vi "write default value String.vi"(8 "error in":errorcluster, 10 "default value":string, 11 "system tag in":refnum<class "tag descriptor.lvclass">) -> (0 "error out":errorcluster, 3 "system tag out":refnum<class "tag descriptor.lvclass">)   [LabVIEW 2013, in "tag bus.lvlib" / "tag descriptor.lvclass"]
doc: "Converts the provided default value into a string and stores that as the raw default value within the tag."
uses:
  tag descriptor.lvclass
  Data Type.ctl
  tag descriptor.lvclass/tag descriptor.ctl
  tag bus.lvlib
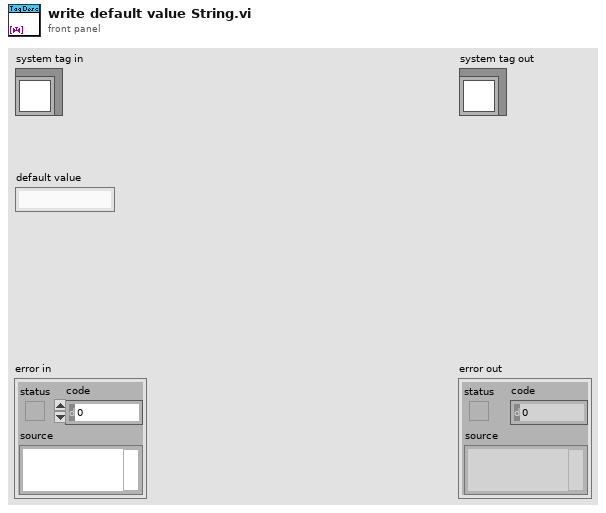
[diagram p1: front panel]
types:
  T1 = typedef "tag bus.lvlib/tag descriptor.lvclass/Data Type.ctl" = enum16{"Double", "Single", "I64", "I32", "I16", "I8", "U64", "U32", "U16", "U8", "Boolean", "String", "Array of Double", "Array of Single", "Array of I64", "Array of I32", "Array of I16", "Array of I8", "Array of U64", "Array of U32", "Array of U16", "Array of U8", "Array of Boolean", "Array of String"}
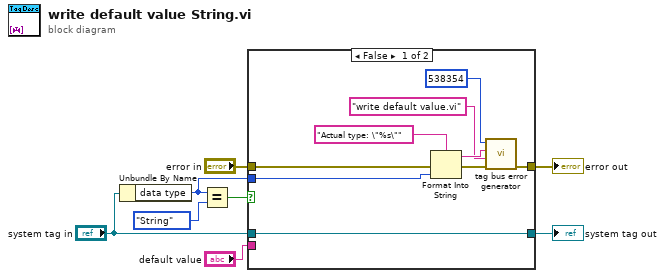
[diagram p0: block diagram]
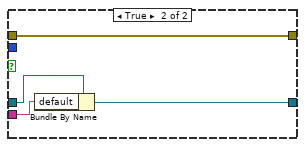
[diagram p2: hidden frame]
diagram:
  n1 = Unbundle By Name("system tag in") -> ("data type"=w4:T1)
  n2 = Equal?(x=w4, y=Data_Type."String") -> (x = y?=w7:bool)
  n3 = case shown="False" w7 {
    tunnel: "error in" -> [w17 w21]
    tunnel: [w13 w21] -> w5
    tunnel: w4 -> [w12 _]
    tunnel: [w10 w19] -> w3
    tunnel: "system tag in" -> [w10 w20]
    tunnel: "default value" -> [_ w18]
    frame False {
      n4 = Format Into String(format string="Actual type: \"%s\"", error in=w17, w12) -> (resulting string=w14:string, error out=w15:errorcluster)  [unwired: 1 in]
      n5 = call "tag bus error generator.vi"("error in"=w15, "source"="write default value.vi", "append error message"=w14, "error code (0)"=538354) -> ("error out"=w13:errorcluster)  [unwired: 5 in]
    }
    frame True {
      n6 = Bundle By Name(cluster=w20, "default"=w18) -> (w19:refnum<class "tag descriptor.lvclass">)
    }
  }
  "error out" <- w5
  "system tag out" <- w3
